vi "waveformpreptesttele.vi"(9 "1762 pulse length (units of .1 us)":dbl) -> (3 "digital waveform out 2":digitalwaveform(waveform)={"t0"=timestamp(0 s since 1904-01-01), "dt"=1e-06, "Y"={"transitions"=[0, 10001], "data"=[[1, 1, 0, 0], [0, 0, 0, 0]]}, "error"={"status"=FALSE, "code"=37421928, "source"=""}})   [LabVIEW 2012]
uses:
  <vilib>/Waveform/DWDTOps.llb/Digital Pattern Generator (Single Value).vi
  <vilib>/Waveform/DWDTOps.llb/DWDT Append Digital Samples.vi
panel:
  out "Mixed Signal Graph":digitalwaveform(graph)
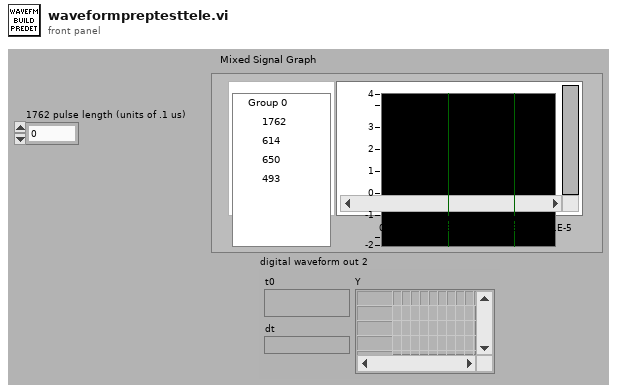
[diagram p1: front panel]
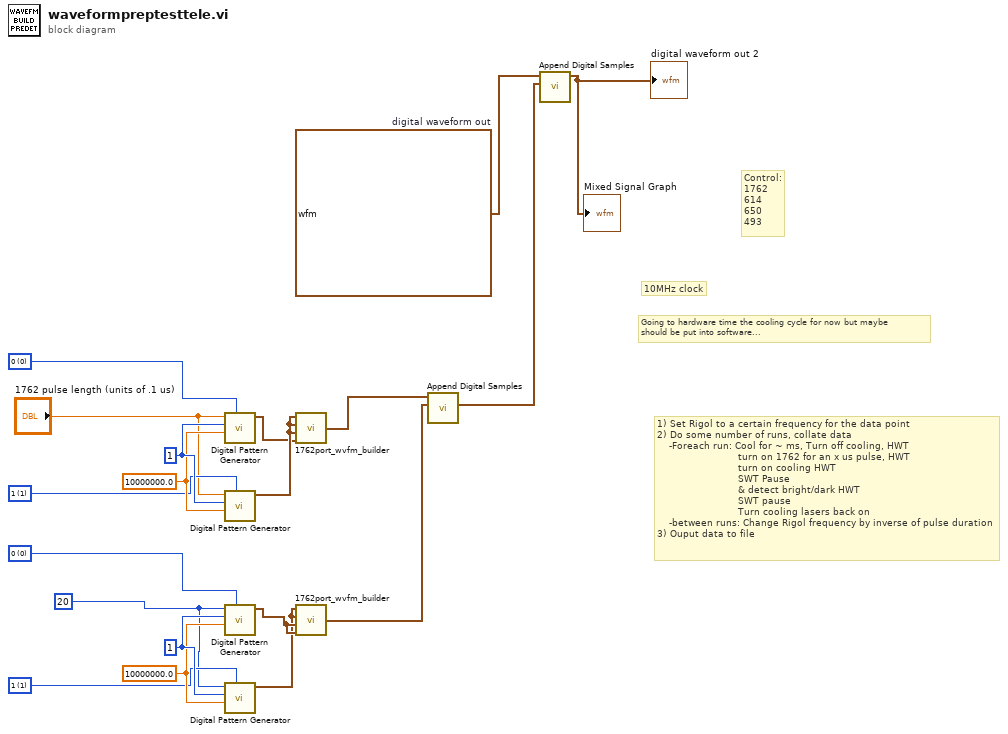
[diagram p0: block diagram]
diagram:
  w1 = u32 20 ("number of samples")
  w8 = u8 0 items=["0", "1", "Z", "L", "H", "X", "T", "V"] ("value")
  w7 = u32 1 ("number of signals")
  w5 = u8 1 items=["0", "1", "Z", "L", "H", "X", "T", "V"] ("value")
  w6 = 10000000.0 ("rate")
  w19 = u8 0 items=["0", "1", "Z", "L", "H", "X", "T", "V"] ("value")
  w18 = u32 1 ("number of signals")
  w16 = u8 1 items=["0", "1", "Z", "L", "H", "X", "T", "V"] ("value")
  w17 = 10000000.0 ("rate")
  w13 = digitalwaveform {"t0"=timestamp(0 s since 1904-01-01), "dt"=1e-07, "Y"={"transitions"=[0, 100, 200, 300], "data"=[[1, 1, 0, 0], [0, 1, 0, 0], [0, 0, 0, 0], [0, 0, 0, 0]]}, "error"={"status"=FALSE, "code"=37421928, "source"=""}}  # digital waveform out
  # "Going to hardware time the cooling cycle for now but maybe\nshould be put into software..."
  # "10MHz clock"
  # "Control:\n1762\n614\n650\n493"
  # "1) Set Rigol to a certain frequency for the data point\n2) Do some number of runs, collate data\n    -Foreach run: Cool for ~ ms, Turn off cooling, HWT\n                           turn on 1762 for an x us pulse, HWT\n                           turn on cooling HWT\n                           SWT Pause\n                           & detect bright/dark HWT\n                           SWT pause\n                           Turn cooling lasers back on \n    -between runs: Change Rigol frequency by inverse of pulse duration\n3) Ouput data to file"
  n1 = call-poly <vilib>:"Digital Pattern Generator.vi"("value"=w19, "sample rate"=w17, "number of signals"=w18, "number of samples"="1762 pulse length (units of .1 us)") -> ("digital waveform"=w9:digitalwaveform)  [unwired: 6 in, 1 out]
  n2 = call-poly <vilib>:"Digital Pattern Generator.vi"("value"=w16, "sample rate"=w17, "number of signals"=w18, "number of samples"="1762 pulse length (units of .1 us)") -> ("digital waveform"=w10:digitalwaveform)  [unwired: 6 in, 1 out]
  n3 = call-poly <vilib>:"Digital Pattern Generator.vi"("value"=w8, "sample rate"=w6, "number of signals"=w7, "number of samples"=w1) -> ("digital waveform"=w3:digitalwaveform)  [unwired: 6 in, 1 out]
  n4 = call-poly <vilib>:"Digital Pattern Generator.vi"("value"=w5, "sample rate"=w6, "number of signals"=w7, "number of samples"=w1) -> ("digital waveform"=w2:digitalwaveform)  [unwired: 6 in, 1 out]
  n5 = call "1762port_wvfm_builder.vi"("614"=w9, "1762"=w10, "650"=w10, "493"=w10) -> ("out"=w11:digitalwaveform)
  n6 = call "1762port_wvfm_builder.vi"("614"=w3, "1762"=w3, "650"=w2, "493"=w2) -> ("out"=w4:digitalwaveform)
  n7 = call-poly <vilib>:"Append Digital Samples.vi"("digital waveform B"=w4, "digital waveform A"=w11) -> ("digital waveform out"=w12:digitalwaveform)  [unwired: 8 in, 1 out]
  n8 = call-poly <vilib>:"Append Digital Samples.vi"("digital waveform B"=w12, "digital waveform A"=w13) -> ("digital waveform out"=→"Mixed Signal Graph" →"digital waveform out 2":digitalwaveform)  [unwired: 8 in, 1 out]
